vi "Generate colour array.vi"(11 "Combo Box":string) -> (3 "Array":u32[](array[numeric]))   [LabVIEW 2015]
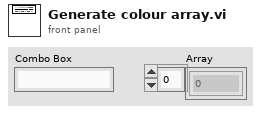
[diagram p1: front panel]
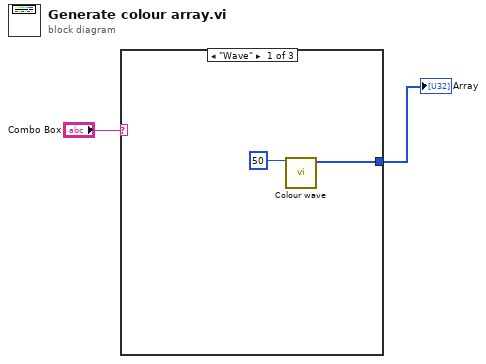
[diagram p0: block diagram]
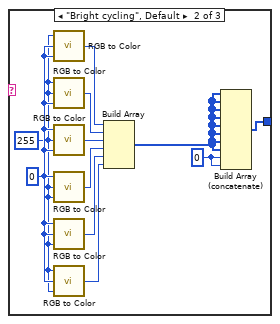
[diagram p2: hidden frame]
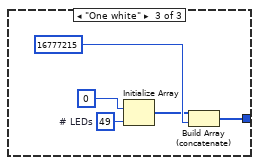
[diagram p3: hidden frame]
diagram:
  n1 = case shown="\"Wave\"" "Combo Box" {
    tunnel: [w4 w6 w16] -> w2
    frame "Wave" {
      n2 = call "Colour wave.vi"("Numeric"=50) -> ("Array"=w4:u32[])  [unwired: 10 in]
    }
    frame "Bright cycling", Default {
      w5 = u32 0 ("Color")
      w11 = u8 0 ("G")
      w10 = u8 255 ("R")
      n3 = call <vilib>:"RGB to Color.vi"("B"=w11, "G"=w11, "R"=w10) -> ("Color"=w7:u32)
      n4 = call <vilib>:"RGB to Color.vi"("B"=w11, "G"=w10, "R"=w10) -> ("Color"=w14:u32)
      n5 = call <vilib>:"RGB to Color.vi"("B"=w11, "G"=w10, "R"=w11) -> ("Color"=w9:u32)
      n6 = call <vilib>:"RGB to Color.vi"("B"=w10, "G"=w10, "R"=w11) -> ("Color"=w13:u32)
      n7 = call <vilib>:"RGB to Color.vi"("B"=w10, "G"=w11, "R"=w11) -> ("Color"=w8:u32)
      n8 = call <vilib>:"RGB to Color.vi"("B"=w10, "G"=w11, "R"=w10) -> ("Color"=w12:u32)
      n9 = Build Array(w7, w14, w9, w13, w8, w12) -> (w15:u32[])
      n10 = Build Array (concatenate)(w15, w15, w15, w15, w15, w15, w15, w15, w5, w5) -> (w6:u32[])
    }
    frame "One white" {
      w17 = 49  # # LEDs
      n11 = Initialize Array(0 ("Color"), w17) -> (w19:i32[])
      n12 = Build Array (concatenate)(w19, u32 16777215 ("Color")) -> (w16:u32[])
    }
  }
  "Array" <- w2
